vi "ManipWaitForPiece.vi"(2 "Reinit":bool, 3 "Parameter String":string) -> (0 "Error Out":errorcluster, 1 "Advance Trigger":bool)   [LabVIEW 2020]
doc: "This VI pauses the drive sequencer until the driver presses the \"advance system check\" button on the joystick, the joystick will rumble while waiting for the button.\n\nParameters:\nNone"
uses:
  SafeParser_Integer.vi
  GlobalGripper.vi
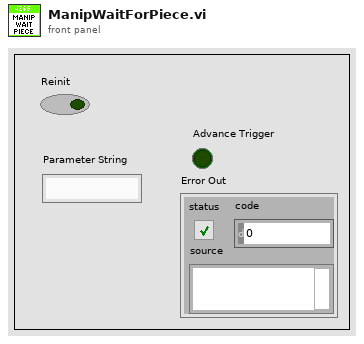
[diagram p1: front panel]
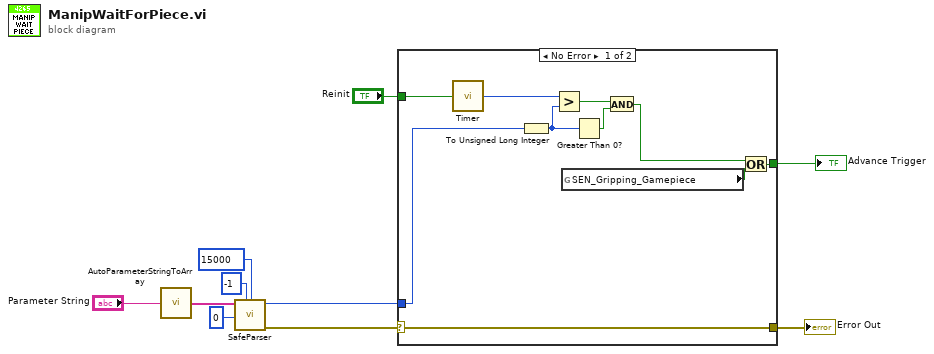
[diagram p0: block diagram]
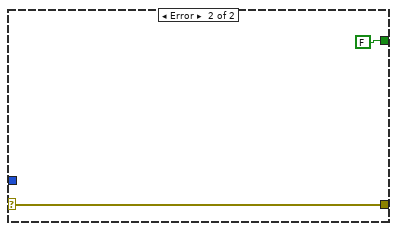
[diagram p2: hidden frame]
diagram:
  n1 = call "AutoParameterStringToArray.vi"("Parameter String"="Parameter String") -> ("Parsed Parameters"=w3:string[])
  n2 = call-poly "SafeParser.vi"("Maximum"=15000, "Minimum"=-1, "Array Index"=0 ("Parameter Index"), "String Array"=w3) -> ("Error Out"=w7:errorcluster, "Typecast  Value"=w8:i32)  [unwired: 6 in]
  n3 = case shown="No Error" w7 {
    selector: w7 -> [w20 w22]
    tunnel: [w15 FALSE] -> w2
    tunnel: "Reinit" -> [w13 _]
    tunnel: [w20 w22] -> w1
    tunnel: w8 -> [w14 _]
    frame No Error {
      n4 = call "Timer.vi"("Reset Timer"=w13) -> ("Time (ms)"=w12:u32)
      n5 = To Unsigned Long Integer(number=w14) -> (unsigned 32bit integer=w16:u32)
      n6 = Greater?(x=w12, y=w16) -> (0:w19:bool)
      n7 = global read "GlobalGripper.vi" "SEN_Gripping_Gamepiece"() -> (w11:bool)
      n8 = Greater Than 0?(x=w16) -> (x > 0?=w18:bool)
      n9 = And(x=w19, y=w18) -> (x .and. y?=w17:bool)
      n10 = Or(x=w17, y=w11) -> (x .or. y?=w15:bool)
    }
    frame Error {
    }
  }
  "Advance Trigger" <- w2
  "Error Out" <- w1
